vi "sokudo-create.vi"() -> (0 "Sudoku":i32[][](array[numeric]))   [LabVIEW 2014]
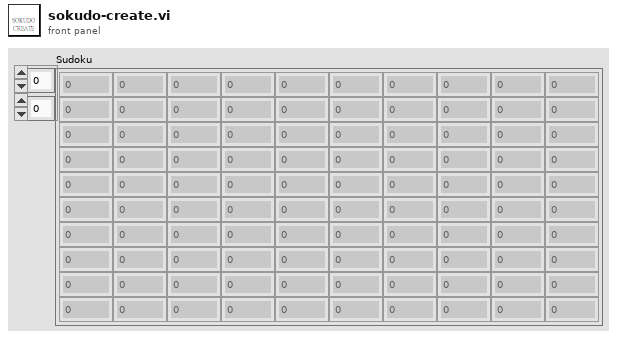
[diagram p1: front panel]
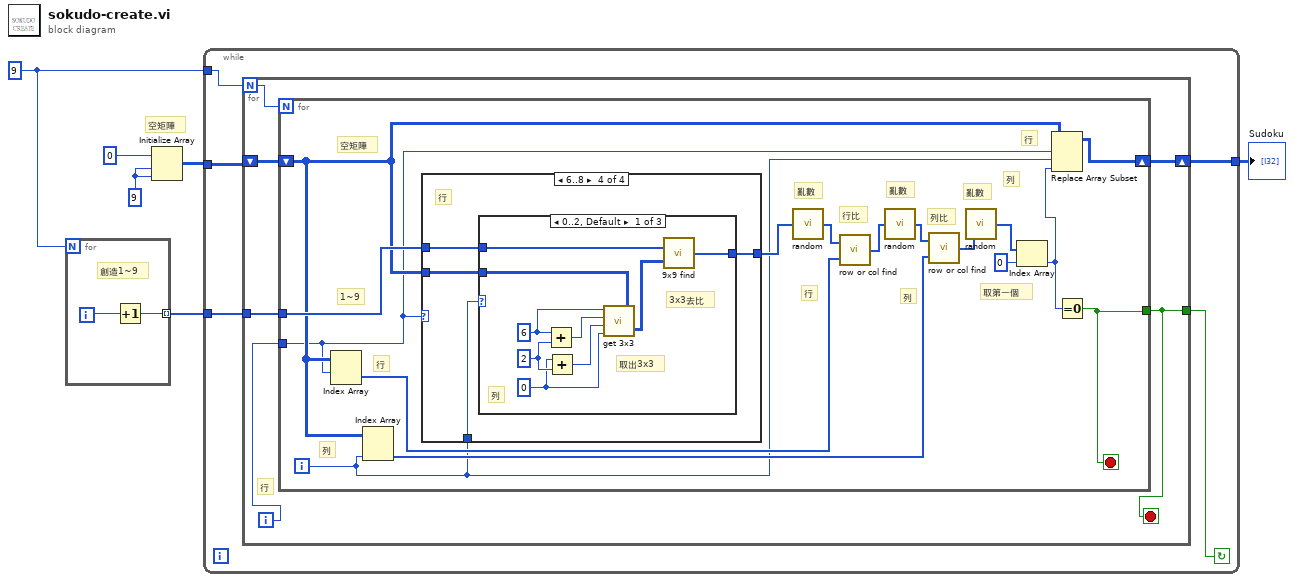
[diagram p0: block diagram]
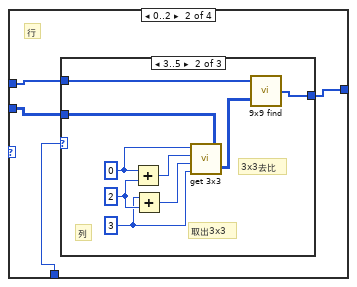
[diagram p3: hidden frame]
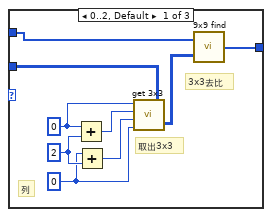
[diagram p4: hidden frame]
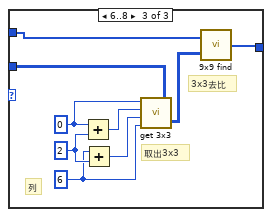
[diagram p5: hidden frame]
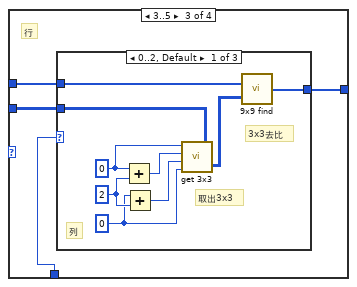
[diagram p6: hidden frame]
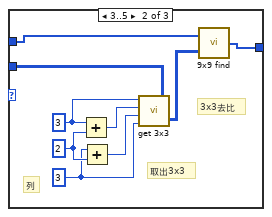
[diagram p7: hidden frame]
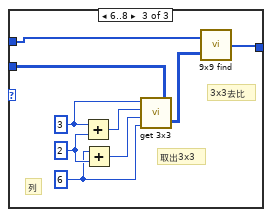
[diagram p8: hidden frame]
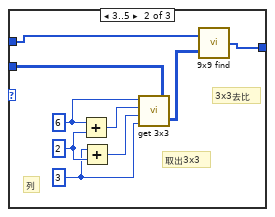
[diagram p9: hidden frame]
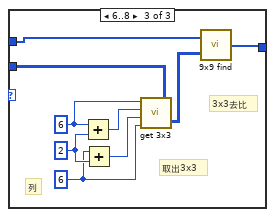
[diagram p10: hidden frame]
diagram:
  w3 = 9
  w5 = 9
  # "空矩陣"
  n1 = for {
    N: w3 -> [_]
    tunnel: [w7] -> w4 mode=indexing
    i -> [w8]
    # "創造1~9"
    n2 = Increment(x=w8) -> (x+1=w7:i32)
  }
  n3 = Initialize Array(0, w5, w5) -> (w2:i32[][])
  n4 = while {
    tunnel: w4 -> [w11]
    tunnel: w3 -> [w13]
    tunnel: w2 -> [w12]
    tunnel: [w9] -> w1
    stop <- w10 continue-if-true
    n5 = for {
      N: w13 -> [w19]
      shift-right: [w17] -> w9
      shift-left: w12 -> [w18]
      tunnel: w11 -> [w16]
      tunnel: [w14] -> w10
      i -> [w15]
      stop <- w14 stop-if-true
      # "行"
      n6 = for {
        N: w19 -> [_]
        shift-right: [w23] -> w17
        shift-left: w18 -> [w25]
        tunnel: w16 -> [w35]
        tunnel: w15 -> [w24]
        tunnel: [w21] -> w14
        i -> [w20]
        stop <- w21 stop-if-true
        # "列比"
        # "行比"
        # "亂數"
        # "亂數"
        # "亂數"
        # "1~9"
        # "空矩陣"
        # "取第一個"
        # "列"
        # "行"
        # "行"
        # "列"
        # "行"
        # "列"
        n7 = Index Array(array=w25, index (row)=w24) -> (element=w28:i32[])  [unwired: 1 in]
        n8 = Index Array(array=w25, index (col)=w20) -> (element=w29:i32[])  [unwired: 1 in]
        n9 = case shown="6..8" w24 {
          tunnel: w35 -> [w36 w40 w71 w100]
          tunnel: w25 -> [_ w39 w70 w101]
          tunnel: w20 -> [_ w37 w68 w99]
          tunnel: [w36 w38 w69 w102] -> w34
          frame 10, Default {
          }
          frame 0..2 {
            # "行"
            n10 = case shown="3..5" w37 {
              tunnel: [w48 w52 w61] -> w38
              tunnel: w39 -> [w42 w51 w60]
              tunnel: w40 -> [w41 w50 w59]
              frame 0..2, Default {
                w47 = 2 ("y")
                w43 = 0 ("Col 1")
                w46 = 0 ("Row 1")
                # "3x3去比"
                # "取出3x3"
                # "列"
                n11 = Add(x=w46, y=w47) -> (x+y=w45:i32)
                n12 = Add(x=w43, y=w47) -> (x+y=w44:i32)
                n13 = call "get 3x3.vi"("input"=w42, "COL 2"=w43, "COL 1"=w44, "ROW 2"=w45, "ROW 1"=w46) -> ("output"=w49:i32[][])
                n14 = call "9x9 find.vi"("9x9  input"=w49, "1~9 input"=w41) -> ("1~9  output"=w48:i32[])
              }
              frame 3..5 {
                w57 = 2 ("y")
                w53 = 3 ("Col 1")
                w56 = 0 ("Row 1")
                # "3x3去比"
                # "取出3x3"
                # "列"
                n15 = Add(x=w56, y=w57) -> (x+y=w55:i32)
                n16 = Add(x=w53, y=w57) -> (x+y=w54:i32)
                n17 = call "get 3x3.vi"("input"=w51, "COL 2"=w53, "COL 1"=w54, "ROW 2"=w55, "ROW 1"=w56) -> ("output"=w58:i32[][])
                n18 = call "9x9 find.vi"("9x9  input"=w58, "1~9 input"=w50) -> ("1~9  output"=w52:i32[])
              }
              frame 6..8 {
                w66 = 2 ("y")
                w62 = 6 ("Col 1")
                w65 = 0 ("Row 1")
                # "3x3去比"
                # "取出3x3"
                # "列"
                n19 = Add(x=w65, y=w66) -> (x+y=w64:i32)
                n20 = Add(x=w62, y=w66) -> (x+y=w63:i32)
                n21 = call "get 3x3.vi"("input"=w60, "COL 2"=w62, "COL 1"=w63, "ROW 2"=w64, "ROW 1"=w65) -> ("output"=w67:i32[][])
                n22 = call "9x9 find.vi"("9x9  input"=w67, "1~9 input"=w59) -> ("1~9  output"=w61:i32[])
              }
            }
          }
          frame 3..5 {
            # "行"
            n23 = case shown="0..2, Default" w68 {
              tunnel: [w79 w83 w92] -> w69
              tunnel: w70 -> [w73 w81 w90]
              tunnel: w71 -> [w72 w82 w91]
              frame 0..2, Default {
                w78 = 2 ("y")
                w74 = 0 ("Col 1")
                w77 = 0 ("Row 1")
                # "3x3去比"
                # "取出3x3"
                # "列"
                n24 = Add(x=w77, y=w78) -> (x+y=w76:i32)
                n25 = Add(x=w74, y=w78) -> (x+y=w75:i32)
                n26 = call "get 3x3.vi"("input"=w73, "COL 2"=w74, "COL 1"=w75, "ROW 2"=w76, "ROW 1"=w77) -> ("output"=w80:i32[][])
                n27 = call "9x9 find.vi"("9x9  input"=w80, "1~9 input"=w72) -> ("1~9  output"=w79:i32[])
              }
              frame 3..5 {
                w88 = 2 ("y")
                w84 = 3 ("Col 1")
                w87 = 3 ("Row 1")
                # "3x3去比"
                # "取出3x3"
                # "列"
                n28 = Add(x=w87, y=w88) -> (x+y=w86:i32)
                n29 = Add(x=w84, y=w88) -> (x+y=w85:i32)
                n30 = call "get 3x3.vi"("input"=w81, "COL 2"=w84, "COL 1"=w85, "ROW 2"=w86, "ROW 1"=w87) -> ("output"=w89:i32[][])
                n31 = call "9x9 find.vi"("9x9  input"=w89, "1~9 input"=w82) -> ("1~9  output"=w83:i32[])
              }
              frame 6..8 {
                w97 = 2 ("y")
                w93 = 6 ("Col 1")
                w96 = 3 ("Row 1")
                # "3x3去比"
                # "取出3x3"
                # "列"
                n32 = Add(x=w96, y=w97) -> (x+y=w95:i32)
                n33 = Add(x=w93, y=w97) -> (x+y=w94:i32)
                n34 = call "get 3x3.vi"("input"=w90, "COL 2"=w93, "COL 1"=w94, "ROW 2"=w95, "ROW 1"=w96) -> ("output"=w98:i32[][])
                n35 = call "9x9 find.vi"("9x9  input"=w98, "1~9 input"=w91) -> ("1~9  output"=w92:i32[])
              }
            }
          }
          frame 6..8 {
            # "行"
            n36 = case shown="0..2, Default" w99 {
              tunnel: [w110 w114 w123] -> w102
              tunnel: w101 -> [w104 w112 w121]
              tunnel: w100 -> [w103 w113 w122]
              frame 0..2, Default {
                w109 = 2 ("y")
                w105 = 0 ("Col 1")
                w108 = 6 ("Row 1")
                # "3x3去比"
                # "取出3x3"
                # "列"
                n37 = Add(x=w108, y=w109) -> (x+y=w107:i32)
                n38 = Add(x=w105, y=w109) -> (x+y=w106:i32)
                n39 = call "get 3x3.vi"("input"=w104, "COL 2"=w105, "COL 1"=w106, "ROW 2"=w107, "ROW 1"=w108) -> ("output"=w111:i32[][])
                n40 = call "9x9 find.vi"("9x9  input"=w111, "1~9 input"=w103) -> ("1~9  output"=w110:i32[])
              }
              frame 3..5 {
                w119 = 2 ("y")
                w115 = 3 ("Col 1")
                w118 = 6 ("Row 1")
                # "3x3去比"
                # "取出3x3"
                # "列"
                n41 = Add(x=w118, y=w119) -> (x+y=w117:i32)
                n42 = Add(x=w115, y=w119) -> (x+y=w116:i32)
                n43 = call "get 3x3.vi"("input"=w112, "COL 2"=w115, "COL 1"=w116, "ROW 2"=w117, "ROW 1"=w118) -> ("output"=w120:i32[][])
                n44 = call "9x9 find.vi"("9x9  input"=w120, "1~9 input"=w113) -> ("1~9  output"=w114:i32[])
              }
              frame 6..8 {
                w128 = 2 ("y")
                w124 = 6 ("Col 1")
                w127 = 6 ("Row 1")
                # "3x3去比"
                # "取出3x3"
                # "列"
                n45 = Add(x=w127, y=w128) -> (x+y=w126:i32)
                n46 = Add(x=w124, y=w128) -> (x+y=w125:i32)
                n47 = call "get 3x3.vi"("input"=w121, "COL 2"=w124, "COL 1"=w125, "ROW 2"=w126, "ROW 1"=w127) -> ("output"=w129:i32[][])
                n48 = call "9x9 find.vi"("9x9  input"=w129, "1~9 input"=w122) -> ("1~9  output"=w123:i32[])
              }
            }
          }
        }
        n49 = call "random.vi"("Input"=w34) -> ("output"=w33:i32[])
        n50 = call "row or col find.vi"("row or col"=w28, "1~9 input"=w33) -> ("1~9 output"=w32:i32[])
        n51 = call "random.vi"("Input"=w32) -> ("output"=w31:i32[])
        n52 = call "row or col find.vi"("row or col"=w29, "1~9 input"=w31) -> ("1~9 output"=w30:i32[])
        n53 = call "random.vi"("Input"=w30) -> ("output"=w27:i32[])
        n54 = Index Array(array=w27, index=0) -> (element=w22:i32)
        n55 = Replace Array Subset(array=w25, new element=w22, index (row)=w24, index (col)=w20) -> (w23:i32[][])
        n56 = Equal To 0?(x=w22) -> (x = 0?=w21:bool)
      }
    }
  }
  "Sudoku" <- w1
